vi "_read_from_port.vi"(0 "Serial port in":refnum<visa-resource-name>, 1 "Number of bytes to read (0)":u32, 3 "error in (no error)":errorcluster) -> (7 "Serial port out":refnum<visa-resource-name>, 8 "Read buffer":string, 9 "Number of bytes read":u32, 10 "error out":errorcluster)   [LabVIEW 2016, in "Chemyx_Syringe_Pump_driver.lvlib"]
doc: "Reads number of bytes from serial port in. If number of bytes is 0 (default), reads all available bytes. Result is outpu to read buffer. Serial port out duplicate Serial port in."
uses:
  Chemyx_Syringe_Pump_driver.lvlib
  <vilib>/Utility/error.llb/Error Cluster From Error Code.vi
  <vilib>/ErrorRing/Error Ring.xnode
panel:
  # "Reads number of bytes from serial port in. If number of bytes is 0 (default), reads all available bytes. Result is outpu to read buffer. Serial port out duplicate Serial port in."
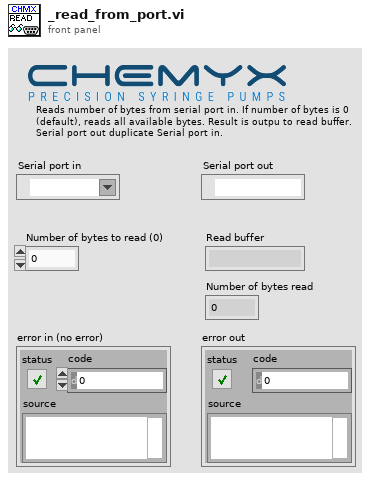
[diagram p1: front panel]
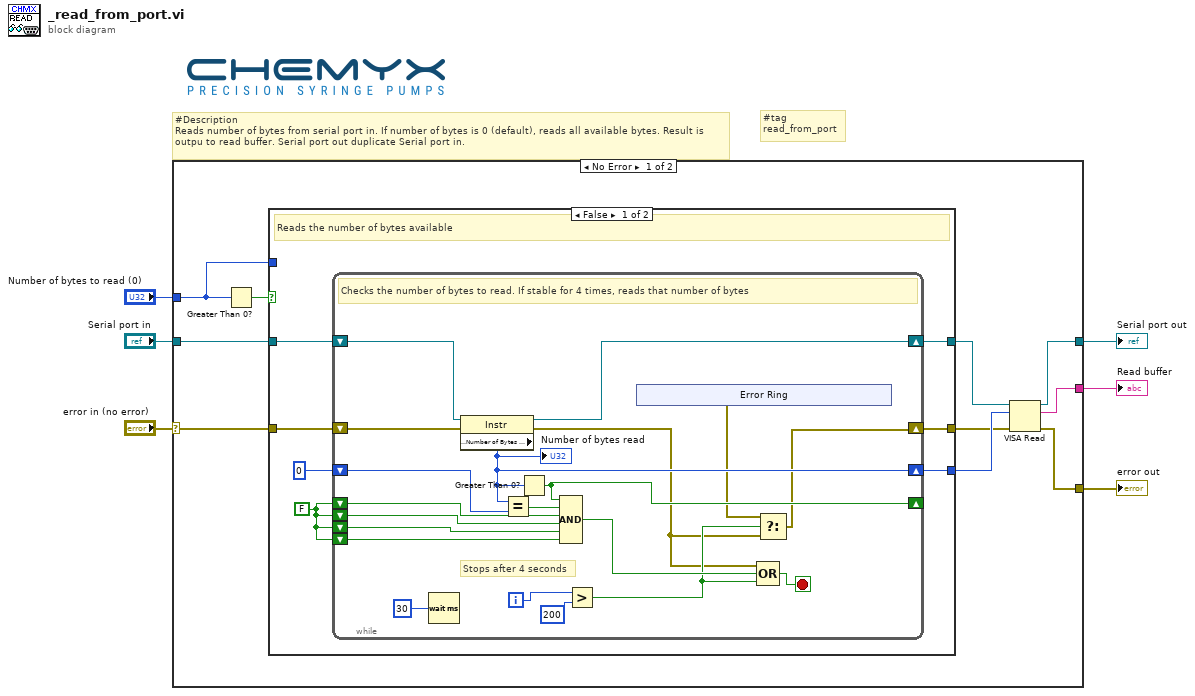
[diagram p0: block diagram]
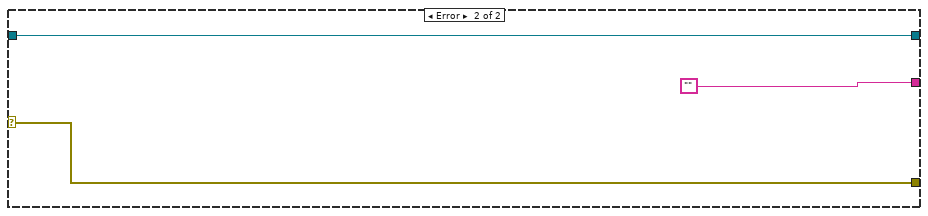
[diagram p3: hidden frame]
diagram:
  # "#tag\nread_from_port"
  # "#Description\nReads number of bytes from serial port in. If number of bytes is 0 (default), reads all available bytes. Result is outpu to read buffer. Serial port out duplicate Serial port in."
  n1 = case shown="No Error" "error in (no error)" {
    selector: "error in (no error)" -> [w7 w52]
    tunnel: "Serial port in" -> [w14 w53]
    tunnel: [w12 w53] -> w5
    tunnel: [w11 w52] -> w4
    tunnel: [w10 ""] -> w3
    tunnel: "Number of bytes to read (0)" -> [w8 _]
    frame No Error {
      n2 = Greater Than 0?(x=w8) -> (x > 0?=w9:bool)
      n3 = case shown="False" w9 {
        tunnel: [w23 w50] -> w16
        tunnel: [w22 w48] -> w15
        tunnel: w14 -> [w21 w48]
        tunnel: [w20 w49] -> w13
        tunnel: w7 -> [w19 w49]
        tunnel: w8 -> [_ w50]
        frame False {
          w18 = FALSE
          # "Reads the number of bytes available"
          n4 = while {
            shift-right: [w24] -> w20
            shift-left: w19 -> [w43]
            shift-right: [w41] -> w22
            shift-left: w21 -> [w42]
            shift-right: [w34] -> _
            shift-left: w18 -> [w32]
            shift-left: w18 -> [w31]
            shift-left: w18 -> [w30]
            shift-left: w18 -> [w39]
            shift-right: [w35] -> w23
            shift-left: u32 0 -> [w36]
            i -> [w29]
            stop <- w33 stop-if-true
            # "Stops after 4 seconds"
            # "Checks the number of bytes to read. If stable for 4 times, reads that number of bytes"
            n5 = Wait (ms)(milliseconds to wait=u32 30) -> ()  [unwired: 1 out]
            n6 = property class="Instr"(reference=w42, error in=w43) -> (reference out=w41:refnum<visa-resource-name>, error out=w26:errorcluster, "Serial Settings:Number of Bytes at Serial Port"=w35:u32)
            "Number of bytes read" <- w35
            n7 = Equal?(x=w35, y=w36) -> (x = y?=w37:bool)
            n8 = Greater Than 0?(x=w35) -> (x > 0?=w34:bool)
            n9 = Compound Arithmetic op=AND(w34, w37, w39, w32, w31, w30) -> (w38:bool)
            n10 = Greater?(x=w29, y=200) -> (0:w27:bool)
            n11 = xnode "Error Ring"() -> ("error out"=w25:errorcluster)
            n12 = Compound Arithmetic op=OR(w26, w38, w27) -> (w33:bool)
            n13 = Select(t=w25, s=w27, f=w26) -> (s? t:f=w24:errorcluster)
          }
        }
        frame True {
          # "Reads the number of bytes provided"
        }
      }
      n14 = VISA Read(VISA resource name=w15, byte count=w16, error in (no error)=w13) -> (VISA resource name out=w12:refnum<visa-resource-name>, read buffer=w10:string, error out=w11:errorcluster)  [unwired: 1 out]
    }
    frame Error {
    }
  }
  "Serial port out" <- w5
  "error out" <- w4
  "Read buffer" <- w3
